vi "Lock Control AE v2.vi"(1 "Lock Control  in":T1, 2 "Action":T2) -> (0 "Lock Control  out":T1)   [LabVIEW 2014]
uses:
  Controls/Standard Action for Focus Lock.ctl
  Controls/Focus Lock.ctl
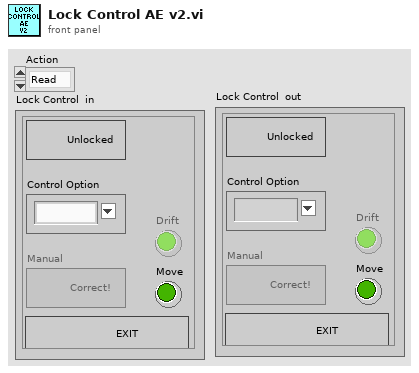
[diagram p1: front panel]
types:
  T1 = typedef "Focus Lock.ctl" = cluster{"EXIT":bool, "Lock Current":bool, "Manual":bool, "Drift":bool, "Move":bool, "Control Option":string}
  T2 = typedef "Standard Action for Focus Lock.ctl" = enum16{"Read", "Write"}
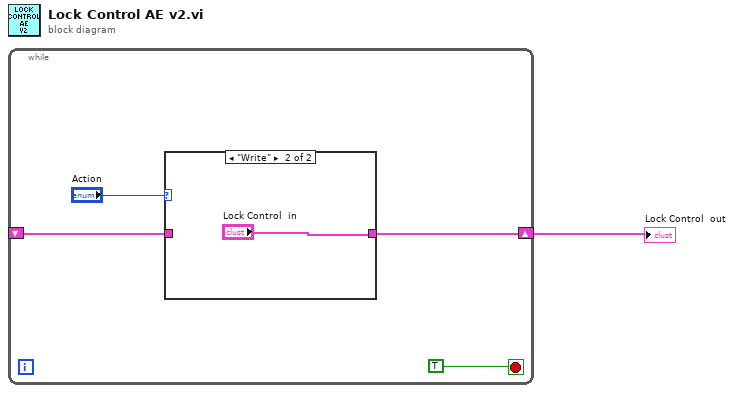
[diagram p0: block diagram]
diagram:
  n1 = while {
    shift-right: [w5] -> w1
    shift-left: _ -> [w4]
    stop <- TRUE stop-if-true
    n2 = case shown="\"Write\"" "Action" {
      tunnel: [w6 "Lock Control  in"] -> w5
      tunnel: w4 -> [w6 _]
      frame "Read", Default {
      }
      frame "Write" {
      }
    }
  }
  "Lock Control  out" <- w1
